vi "Index Array.vi"() -> ()   [LabVIEW 2016]
panel:
  out "Element":dbl
  in  "Index":dbl
  in  "Array":dbl[](array[numeric])
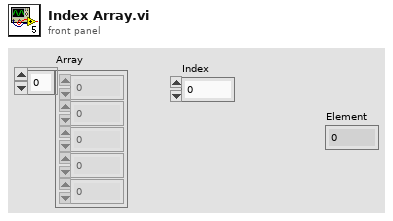
[diagram p1: front panel]
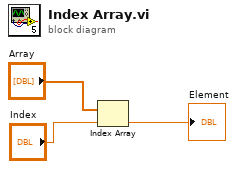
[diagram p0: block diagram]
diagram:
  n1 = Index Array(array="Array", index="Index") -> (element=→"Element":dbl)
